vi "Remove Child.vi"(8 "error in (no error)":errorcluster, 10 "child name":string, 11 "[MDI] Parent in":refnum<class "[MDI] Parent.lvclass">) -> (0 "error out":errorcluster, 3 "[MDI] Parent out":refnum<class "[MDI] Parent.lvclass">)   [LabVIEW 2020, in "[MDI] Parent.lvlib" / "[MDI] Parent.lvclass"]
uses:
  [MDI] Parent.lvclass
  [MDI] Parent.lvclass/[MDI] Parent.ctl
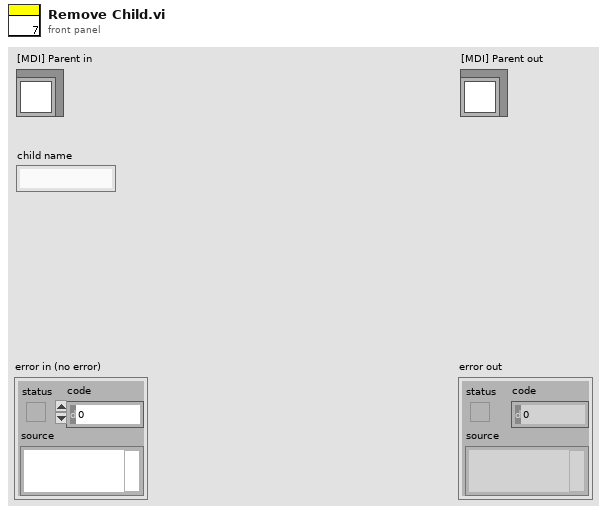
[diagram p1: front panel]
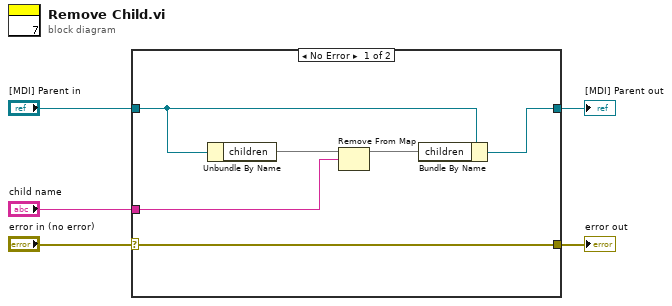
[diagram p0: block diagram]
diagram:
  n1 = case shown="No Error" "error in (no error)" {
    selector: "error in (no error)" -> [w11 w13]
    tunnel: [w11 w13] -> w4
    tunnel: [w7 w12] -> w2
    tunnel: "[MDI] Parent in" -> [w9 w12]
    tunnel: "child name" -> [w6 _]
    frame No Error {
      n2 = Unbundle By Name(w9) -> ("children"=w10:map{string, refnum<vi>})
      n3 = Remove From Map(10:w6, 11:w10) -> (3:w8:map{string, refnum<vi>})  [unwired: 2 out]
      n4 = Bundle By Name(cluster=w9, "children"=w8) -> (w7:refnum<class "[MDI] Parent.lvclass">)
    }
    frame Error {
    }
  }
  "error out" <- w4
  "[MDI] Parent out" <- w2
